vi "Write Data.vi"(10 "Data":i32, 11 "Game State Task Msg in":refnum<class "Game State Task Msg.lvclass">) -> (3 "Game State Task Msg out":refnum<class "Game State Task Msg.lvclass">)   [LabVIEW 2021, in "Game State Actor.lvlib" / "Game State Task Msg.lvclass"]
uses:
  Game State Task Msg.lvclass
  Game State Task Msg.lvclass/Game State Task Msg.ctl
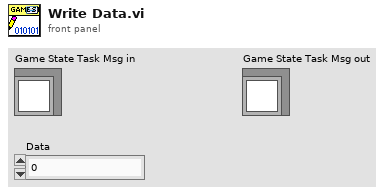
[diagram p1: front panel]
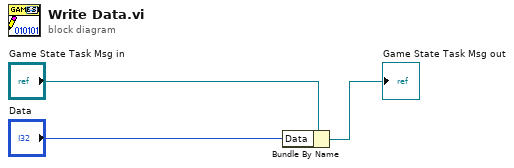
[diagram p0: block diagram]
diagram:
  n1 = Bundle By Name(cluster="Game State Task Msg in", "Data"="Data") -> (→"Game State Task Msg out":refnum<class "Game State Task Msg.lvclass">)
